vi "Charger_Command Write.vi"(6 "error in":errorcluster, 8 "Command":T2(ring)=enum."Enable", 9 "Charger":T1={"address"="COM13", "position"=0, "setpoint"=7500.0} {"setpoint" min=0.0 max=20000.0 step=100.0; "position" min=0 max=5 step=1}) -> (0 "error out":errorcluster, 4 "serial cmd":string)   [LabVIEW 2020]
uses:
  Charger_Input Control.ctl
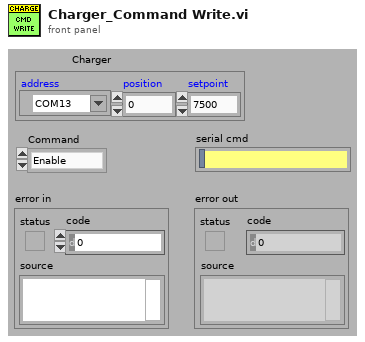
[diagram p1: front panel]
types:
  T1 = typedef "Charger_Input Control.ctl" = cluster{"address":refnum<visa-resource-name>, "position":i32, "setpoint":dbl}
  T2 = enum16{"Disable", "Enable", "Update", "Get Info"}
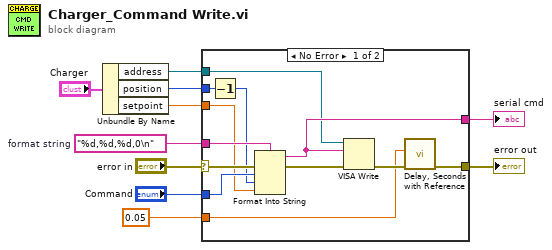
[diagram p0: block diagram]
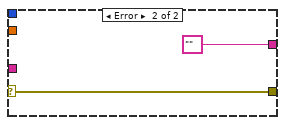
[diagram p2: hidden frame]
diagram:
  w10 = "%d,%d,%d,0\n"  # format string
  n1 = Unbundle By Name("Charger") -> ("address"=w3:refnum<visa-resource-name>, "position"=w2:i32, "setpoint"=w1:dbl)
  n2 = case shown="No Error" "error in" {
    selector: "error in" -> [w16 w24]
    tunnel: w10 -> [w22 _]
    tunnel: [w19 ""] -> w9
    tunnel: "Command" -> [w18 _]
    tunnel: [w15 w24] -> w7
    tunnel: dbl[unit] 0.05 ("delay") -> [w17 _]
    tunnel: w3 -> [w14 _]
    tunnel: w2 -> [w13 _]
    tunnel: w1 -> [w12 _]
    frame No Error {
      n3 = Decrement(x=w13) -> (x-1=w11:i32)
      n4 = Format Into String(format string=w22, error in=w16, w18, w11, w12) -> (resulting string=w19:string, error out=w20:errorcluster)  [unwired: 1 in]
      n5 = VISA Write(VISA resource name=w14, write buffer=w19, error in (no error)=w20) -> (error out=w21:errorcluster)  [unwired: 2 out]
      n6 = call "Delay, Seconds with Reference.vi"("error in"=w21, "delay"=w17) -> ("error out"=w15:errorcluster)  [unwired: 4 in, 2 out]
    }
    frame Error {
    }
  }
  "serial cmd" <- w9
  "error out" <- w7
